vi "Stepper Write.vi"(6 "Set Acceleration (0 to disable)":i16, 7 "Stepper #":u8, 8 "error in":errorcluster, 9 "Set Speed (Steps per Second)":i16=100, 10 "# of Steps to Move":i16, 11 "Arduino Resource":T1={"VISA resource"="", "Board Type"=enum."Arduino Uno", "Connection Type"=enum."USB / Serial", "Bytes Per Packet (15)"=15}) -> (0 "error out":errorcluster, 3 "Arduino Resource Out":T1={"VISA resource"="", "Board Type"=enum."Arduino Uno", "Connection Type"=enum."USB / Serial", "Bytes Per Packet (15)"=15})   [LabVIEW 2011, in "LabVIEW Interface for Arduino.lvlib"]
doc: "Specify the speed and number of steps to move the stepper motor. Optionally, specify acceleration in steps per second per second."
uses:
  LabVIEW Interface for Arduino.lvlib
  Private/Type Defs/Arduino Resource.ctl
  Private/Type Defs/Board Type.ctl
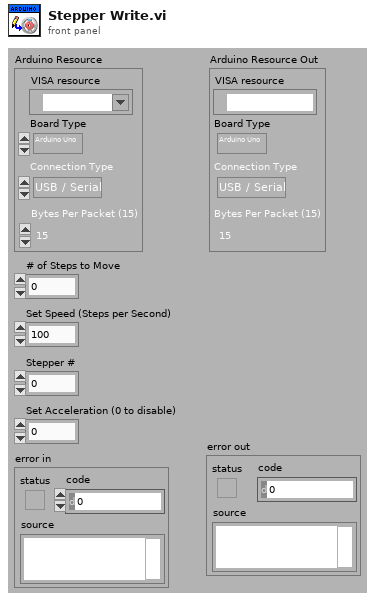
[diagram p1: front panel]
types:
  T1 = typedef "LabVIEW Interface for Arduino.lvlib/Arduino Resource.ctl" = cluster{"VISA resource":refnum<visa-resource-name>, "Board Type":T2, "Connection Type":enum8{"USB / Serial"}, "Bytes Per Packet (15)":u8}
  T2 = typedef "LabVIEW Interface for Arduino.lvlib/Board Type.ctl" = enum16{"Arduino Uno", "Dimuelanove w/Atmega 328", "Mega 2560", "Chipkit Uno32", "Chipkit Max32"}
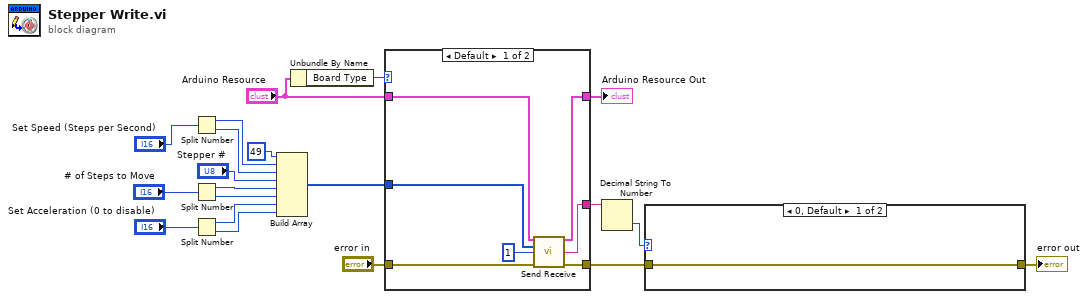
[diagram p0: block diagram]
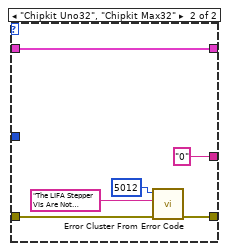
[diagram p2: hidden frame]
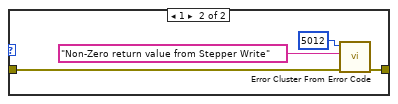
[diagram p3: hidden frame]
diagram:
  n1 = Split Number(x="Set Speed (Steps per Second)") -> (hi(x)=w17:u8, lo(x)=w16:u8)
  n2 = Split Number(x="# of Steps to Move") -> (hi(x)=w14:u8, lo(x)=w13:u8)
  n3 = Split Number(x="Set Acceleration (0 to disable)") -> (hi(x)=w11:u8, lo(x)=w10:u8)
  n4 = Build Array(u8 49, w17, w16, "Stepper #", w14, w13, w11, w10) -> (w5:u8[])
  n5 = Unbundle By Name("Arduino Resource") -> ("Board Type"=w7:T2)
  n6 = case shown="Default" w7 {
    tunnel: "Arduino Resource" -> [w26 w31]
    tunnel: w5 -> [w25 _]
    tunnel: [w24 w31] -> w3
    tunnel: [w23 "0" ("Read Buffer")] -> w4
    tunnel: "error in" -> [w22 w28]
    tunnel: [w21 w29] -> w2
    frame Default {
      n7 = call "Send Receive.vi"("Arduino Resource"=w26, "Data"=w25, "Bytes To Read (0)"=u8 1, "error in"=w22) -> ("Arduino Resource"=w24:T1, "Read Buffer"=w23:string, "error out"=w21:errorcluster)  [unwired: 9 in]
    }
    frame "Chipkit Uno32", "Chipkit Max32" {
      n8 = call <vilib>:"Error Cluster From Error Code.vi"("error in (no error)"=w28, "error message (\"\")"="The LIFA Stepper VIs Are Not Supported On Chipkit Targets." ("source"), "error code (0)"=5012) -> ("error out"=w29:errorcluster)  [unwired: 6 in]
    }
  }
  "Arduino Resource Out" <- w3
  n9 = Decimal String To Number(string=w4) -> (number=w9:i32)  [unwired: 2 in, 1 out]
  n10 = case shown="0, Default" w9 {
    tunnel: w2 -> [w34 w36]
    tunnel: [w34 w35] -> w8
    frame 0, Default {
    }
    frame 1 {
      n11 = call <vilib>:"Error Cluster From Error Code.vi"("error in (no error)"=w36, "error message (\"\")"="Non-Zero return value from Stepper Write" ("source"), "error code (0)"=5012) -> ("error out"=w35:errorcluster)  [unwired: 6 in]
    }
  }
  "error out" <- w8
